vi "Dresden Edit Recipe(in).vi"() -> ()   [LabVIEW 2009] (continued)
                    n1981 = property on="R Single RF Interval length9" class="DigNum (strict)"("DisabledEnum"=w1077) -> ()  [unwired: 2 in, 2 out]
                  }
                }
              }
            }
            n1982 = case shown="False" w984 {
              frame #0 {
                w1926 = 0.0 ("R Cmb Ch2 Step1 Coating Power")
                w1927 = T5."Disabled and Grayed Out" ("Disabled")
                n1983 = local write "R Cmb Ch2 Step1 Coating Power"(w1926) -> ()
                n1984 = local write "R Cmb Ch3 Step1 Coating Power"(w1926) -> ()
                n1985 = local write "R Cmb Interval length 1"(w1926) -> ()
                n1986 = property on="R Cmb Ch3 Step1 Coating Power" class="DigNum (strict)"("DisabledEnum"=w1927) -> ()  [unwired: 2 in, 2 out]
                n1987 = property on="R Cmb Ch2 Step1 Coating Power" class="DigNum (strict)"("DisabledEnum"=w1927) -> ()  [unwired: 2 in, 2 out]
                n1988 = property on="R Cmb Interval length 1" class="DigNum (strict)"("DisabledEnum"=w1927) -> ()  [unwired: 2 in, 2 out]
              }
              frame #1 {
                w1928 = T5."Enabled" ("Disabled")
                n1989 = property on="R Cmb Ch3 Step1 Coating Power" class="DigNum (strict)"("DisabledEnum"=w1928) -> ()  [unwired: 2 in, 2 out]
                n1990 = property on="R Cmb Ch2 Step1 Coating Power" class="DigNum (strict)"("DisabledEnum"=w1928) -> ()  [unwired: 2 in, 2 out]
                n1991 = property on="R Cmb Interval length 1" class="DigNum (strict)"("DisabledEnum"=w1928) -> ()  [unwired: 2 in, 2 out]
              }
            }
            n1992 = case shown="True" "Calculate" {
              frame #0 {
              }
              frame #1 {
                n1993 = stacked-sequence {
                  frame #0 {
                    w1932 = 0.0 ("Lap")
                    n1994 = local read "R Minimum diameter"() -> (w1933:dbl)
                    n1995 = local write "Diameter"(w1933) -> ()
                    n1996 = local write "R  Total length"(w1932) -> ()
                    n1997 = local write "Lap"(w1932) -> ()
                  }
                  frame #1 {
                    n1998 = while {
                      stop <- w1936 stop-if-true
                      n1999 = local read "R Web thickness"() -> (w1946:dbl)
                      n2000 = Wait Until Next ms Multiple(millisecond multiple=u32 10) -> ()  [unwired: 1 out]
                      n2001 = Multiply(x=w1946, y=0.002) -> (x*y=w1945:dbl)
                      n2002 = local read "Lap"() -> (w1949:dbl)
                      n2003 = Increment(x=w1949) -> (x+1=→"Lap":dbl)
                      n2004 = Add(x="Diameter", y=w1945) -> (x+y=w1944:dbl)
                      n2005 = local write "Diameter"(w1944) -> ()
                      n2006 = local read "R Maximum diameter"() -> (w1937:dbl)
                      n2007 = local read "Diameter"() -> (w1934:dbl)
                      n2008 = Greater Or Equal?(x=w1934, y=w1937) -> (x >= y?=w1936:bool)
                      n2009 = local read "R  Total length"() -> (w1935:dbl)
                      n2010 = Multiply(x=w1934, y=3.141592653589793) -> (x*y=w1943:dbl)
                      n2011 = Divide(x=w1943, y=10.0) -> (x/y=w1940:dbl)
                      n2012 = Add(x=w1940, y=w1935) -> (x+y=→"R  Total length":dbl)
                    }
                  }
                }
              }
            }
            n2013 = case shown="False" "Power_single_rf_list_open" {
              frame #0 {
                n2014 = property on="Single_RF_power_power_tab" class="TabCtl (strict)"("Visible"=FALSE) -> ()  [unwired: 2 in, 2 out]
              }
              frame #1 {
                n2015 = property on="Single_RF_power_power_tab" class="TabCtl (strict)"("Visible"=TRUE) -> ()  [unwired: 2 in, 2 out]
              }
            }
            n2016 = local read "R Cmb Step6 Coating Power Active"() -> (w827:bool)
            n2017 = local read "R Cmb Step5 Coating Power Active"() -> (w828:bool)
            n2018 = local read "R Cmb Step7 Coating Power Active"() -> (w826:bool)
            n2019 = case shown="23" "R_Single RF_Mat_sel" {
              frame #0 {
              }
              frame #1 {
                n2020 = local write "R Single RF Target material"("Ag" ("R DC Target material")) -> ()
              }
              frame #2 {
                n2021 = local write "R Single RF Target material"("AgBr" ("R DC Target material")) -> ()
              }
              frame #3 {
                n2022 = local write "R Single RF Target material"("AgCl" ("R DC Target material")) -> ()
              }
              frame #4 {
                n2023 = local write "R Single RF Target material"("Al" ("R DC Target material")) -> ()
              }
              frame #5 {
                n2024 = local write "R Single RF Target material"("Al2O3" ("R DC Target material")) -> ()
              }
              frame #6 {
                n2025 = local write "R Single RF Target material"("As" ("R DC Target material")) -> ()
              }
              frame #7 {
                n2026 = local write "R Single RF Target material"("Au" ("R DC Target material")) -> ()
              }
              frame #8 {
                n2027 = local write "R Single RF Target material"("B" ("R DC Target material")) -> ()
              }
              frame #9 {
                n2028 = local write "R Single RF Target material"("Ba" ("R DC Target material")) -> ()
              }
              frame #10 {
                n2029 = local write "R Single RF Target material"("Be" ("R DC Target material")) -> ()
              }
              frame #11 {
                n2030 = local write "R Single RF Target material"("Bi" ("R DC Target material")) -> ()
              }
              frame #12 {
                n2031 = local write "R Single RF Target material"("Bi2O3" ("R DC Target material")) -> ()
              }
              frame #13 {
                n2032 = local write "R Single RF Target material"("C (Diamond)" ("R DC Target material")) -> ()
              }
              frame #14 {
                n2033 = local write "R Single RF Target material"("C (Graphite)" ("R DC Target material")) -> ()
              }
              frame #15 {
                n2034 = local write "R Single RF Target material"("Ca" ("R DC Target material")) -> ()
              }
              frame #16 {
                n2035 = local write "R Single RF Target material"("CaF" ("R DC Target material")) -> ()
              }
              frame #17 {
                n2036 = local write "R Single RF Target material"("Cd" ("R DC Target material")) -> ()
              }
              frame #18 {
                n2037 = local write "R Single RF Target material"("CdS" ("R DC Target material")) -> ()
              }
              frame #19 {
                n2038 = local write "R Single RF Target material"("CdSe" ("R DC Target material")) -> ()
              }
              frame #20 {
                n2039 = local write "R Single RF Target material"("CdTe" ("R DC Target material")) -> ()
              }
              frame #21 {
                n2040 = local write "R Single RF Target material"("CeF3" ("R DC Target material")) -> ()
              }
              frame #22 {
                n2041 = local write "R Single RF Target material"("CeO" ("R DC Target material")) -> ()
              }
              frame #23 {
                n2042 = local write "R Single RF Target material"("Cr" ("R DC Target material")) -> ()
              }
              frame #24 {
                n2043 = local write "R Single RF Target material"("Cr2O3" ("R DC Target material")) -> ()
              }
              frame #25 {
                n2044 = local write "R Single RF Target material"("Co" ("R DC Target material")) -> ()
              }
              frame #26 {
                n2045 = local write "R Single RF Target material"("Cu" ("R DC Target material")) -> ()
              }
              frame #27 {
                n2046 = local write "R Single RF Target material"("Cu2S (A)" ("R DC Target material")) -> ()
              }
              frame #28 {
                n2047 = local write "R Single RF Target material"("Cu2S (B)" ("R DC Target material")) -> ()
              }
              frame #29 {
                n2048 = local write "R Single RF Target material"("CuS" ("R DC Target material")) -> ()
              }
              frame #30 {
                n2049 = local write "R Single RF Target material"("Dy" ("R DC Target material")) -> ()
              }
              frame #31 {
                n2050 = local write "R Single RF Target material"("Er" ("R DC Target material")) -> ()
              }
              frame #32 {
                n2051 = local write "R Single RF Target material"("Fe" ("R DC Target material")) -> ()
              }
              frame #33 {
                n2052 = local write "R Single RF Target material"("Ga" ("R DC Target material")) -> ()
              }
              frame #34 {
                n2053 = local write "R Single RF Target material"("GaAs" ("R DC Target material")) -> ()
              }
              frame #35 {
                n2054 = local write "R Single RF Target material"("Gd" ("R DC Target material")) -> ()
              }
              frame #36 {
                n2055 = local write "R Single RF Target material"("Ge" ("R DC Target material")) -> ()
              }
              frame #37 {
                n2056 = local write "R Single RF Target material"("Hf" ("R DC Target material")) -> ()
              }
              frame #38 {
                n2057 = local write "R Single RF Target material"("HfO2" ("R DC Target material")) -> ()
              }
              frame #39 {
                n2058 = local write "R Single RF Target material"("Hg" ("R DC Target material")) -> ()
              }
              frame #40 {
                n2059 = local write "R Single RF Target material"("Ho" ("R DC Target material")) -> ()
              }
              frame #41 {
                n2060 = local write "R Single RF Target material"("In" ("R DC Target material")) -> ()
              }
              frame #42 {
                n2061 = local write "R Single RF Target material"("InSb" ("R DC Target material")) -> ()
              }
              frame #43 {
                n2062 = local write "R Single RF Target material"("In2O3" ("R DC Target material")) -> ()
              }
              frame #44 {
                n2063 = local write "R Single RF Target material"("Ir" ("R DC Target material")) -> ()
              }
              frame #45 {
                n2064 = local write "R Single RF Target material"("KCl" ("R DC Target material")) -> ()
              }
              frame #46 {
                n2065 = local write "R Single RF Target material"("La" ("R DC Target material")) -> ()
              }
              frame #47 {
                n2066 = local write "R Single RF Target material"("LaF3" ("R DC Target material")) -> ()
              }
              frame #48 {
                n2067 = local write "R Single RF Target material"("LaO3" ("R DC Target material")) -> ()
              }
              frame #49 {
                n2068 = local write "R Single RF Target material"("Li" ("R DC Target material")) -> ()
              }
              frame #50 {
                n2069 = local write "R Single RF Target material"("LiF" ("R DC Target material")) -> ()
              }
              frame #51 {
                n2070 = local write "R Single RF Target material"("Mg" ("R DC Target material")) -> ()
              }
              frame #52 {
                n2071 = local write "R Single RF Target material"("MgF2" ("R DC Target material")) -> ()
              }
              frame #53 {
                n2072 = local write "R Single RF Target material"("MgO" ("R DC Target material")) -> ()
              }
              frame #54 {
                n2073 = local write "R Single RF Target material"("Mn" ("R DC Target material")) -> ()
              }
              frame #55 {
                n2074 = local write "R Single RF Target material"("MnS" ("R DC Target material")) -> ()
              }
              frame #56 {
                n2075 = local write "R Single RF Target material"("Mo" ("R DC Target material")) -> ()
              }
              frame #57 {
                n2076 = local write "R Single RF Target material"("Na" ("R DC Target material")) -> ()
              }
              frame #58 {
                n2077 = local write "R Single RF Target material"("NaCl" ("R DC Target material")) -> ()
              }
              frame #59 {
                n2078 = local write "R Single RF Target material"("NdF3" ("R DC Target material")) -> ()
              }
              frame #60 {
                n2079 = local write "R Single RF Target material"("Nd2O3" ("R DC Target material")) -> ()
              }
              frame #61 {
                n2080 = local write "R Single RF Target material"("Ni" ("R DC Target material")) -> ()
              }
              frame #62 {
                n2081 = local write "R Single RF Target material"("Nb" ("R DC Target material")) -> ()
              }
              frame #63 {
                n2082 = local write "R Single RF Target material"("Nb2O5" ("R DC Target material")) -> ()
              }
              frame #64 {
                n2083 = local write "R Single RF Target material"("Pb" ("R DC Target material")) -> ()
              }
              frame #65 {
                n2084 = local write "R Single RF Target material"("PbS" ("R DC Target material")) -> ()
              }
              frame #66 {
                n2085 = local write "R Single RF Target material"("Pd" ("R DC Target material")) -> ()
              }
              frame #67 {
                n2086 = local write "R Single RF Target material"("Pt" ("R DC Target material")) -> ()
              }
              frame #68 {
                n2087 = local write "R Single RF Target material"("Re" ("R DC Target material")) -> ()
              }
              frame #69 {
                n2088 = local write "R Single RF Target material"("Rh" ("R DC Target material")) -> ()
              }
              frame #70 {
                n2089 = local write "R Single RF Target material"("Rb" ("R DC Target material")) -> ()
              }
              frame #71 {
                n2090 = local write "R Single RF Target material"("S" ("R DC Target material")) -> ()
              }
              frame #72 {
                n2091 = local write "R Single RF Target material"("Sb" ("R DC Target material")) -> ()
              }
              frame #73 {
                n2092 = local write "R Single RF Target material"("Sc" ("R DC Target material")) -> ()
              }
              frame #74 {
                n2093 = local write "R Single RF Target material"("Se" ("R DC Target material")) -> ()
              }
              frame #75 {
                n2094 = local write "R Single RF Target material"("Si" ("R DC Target material")) -> ()
              }
              frame #76 {
                n2095 = local write "R Single RF Target material"("SiO" ("R DC Target material")) -> ()
              }
              frame #77 {
                n2096 = local write "R Single RF Target material"("SiO2" ("R DC Target material")) -> ()
              }
              frame #78 {
                n2097 = local write "R Single RF Target material"("Sm" ("R DC Target material")) -> ()
              }
              frame #79 {
                n2098 = local write "R Single RF Target material"("Sn" ("R DC Target material")) -> ()
              }
              frame #80 {
                n2099 = local write "R Single RF Target material"("Ta" ("R DC Target material")) -> ()
              }
              frame #81 {
                n2100 = local write "R Single RF Target material"("Ta2O5" ("R DC Target material")) -> ()
              }
              frame #82 {
                n2101 = local write "R Single RF Target material"("Te" ("R DC Target material")) -> ()
              }
              frame #83 {
                n2102 = local write "R Single RF Target material"("Tb" ("R DC Target material")) -> ()
              }
              frame #84 {
                n2103 = local write "R Single RF Target material"("ThF4" ("R DC Target material")) -> ()
              }
              frame #85 {
                n2104 = local write "R Single RF Target material"("Ti" ("R DC Target material")) -> ()
              }
              frame #86 {
                n2105 = local write "R Single RF Target material"("TiO2" ("R DC Target material")) -> ()
              }
              frame #87 {
                n2106 = local write "R Single RF Target material"("TiO" ("R DC Target material")) -> ()
              }
              frame #88 {
                n2107 = local write "R Single RF Target material"("Tl" ("R DC Target material")) -> ()
              }
              frame #89 {
                n2108 = local write "R Single RF Target material"("U" ("R DC Target material")) -> ()
              }
              frame #90 {
                n2109 = local write "R Single RF Target material"("V" ("R DC Target material")) -> ()
              }
              frame #91 {
                n2110 = local write "R Single RF Target material"("W" ("R DC Target material")) -> ()
              }
              frame #92 {
                n2111 = local write "R Single RF Target material"("WC" ("R DC Target material")) -> ()
              }
              frame #93 {
                n2112 = local write "R Single RF Target material"("Y" ("R DC Target material")) -> ()
              }
              frame #94 {
                n2113 = local write "R Single RF Target material"("Y2O3" ("R DC Target material")) -> ()
              }
              frame #95 {
                n2114 = local write "R Single RF Target material"("Yb" ("R DC Target material")) -> ()
              }
              frame #96 {
                n2115 = local write "R Single RF Target material"("Zn" ("R DC Target material")) -> ()
              }
              frame #97 {
                n2116 = local write "R Single RF Target material"("ZnO" ("R DC Target material")) -> ()
              }
              frame #98 {
                n2117 = local write "R Single RF Target material"("ZnSe" ("R DC Target material")) -> ()
              }
              frame #99 {
                n2118 = local write "R Single RF Target material"("ZnS" ("R DC Target material")) -> ()
              }
              frame #100 {
                n2119 = local write "R Single RF Target material"("Zr" ("R DC Target material")) -> ()
              }
              frame #101 {
                n2120 = local write "R Single RF Target material"("ZrO2" ("R DC Target material")) -> ()
              }
              frame #102 {
                n2121 = local write "R Single RF Target material"("Si3N4" ("R DC Target material")) -> ()
              }
              frame #103 {
                n2122 = local write "R Single RF Target material"("ITO" ("R DC Target material")) -> ()
              }
              frame #104 {
                n2123 = local write "R Single RF Target material"("PbI2" ("R DC Target material")) -> ()
              }
            }
            n2124 = case shown="104" "R Cmb Ch3 Mat_sel" {
              frame #0 {
              }
              frame #1 {
                n2125 = local write "R Cmb Ch3 Target material"("Ag" ("R DC Target material")) -> ()
              }
              frame #2 {
                n2126 = local write "R Cmb Ch3 Target material"("AgBr" ("R DC Target material")) -> ()
              }
              frame #3 {
                n2127 = local write "R Cmb Ch3 Target material"("AgCl" ("R DC Target material")) -> ()
              }
              frame #4 {
                n2128 = local write "R Cmb Ch3 Target material"("Al" ("R DC Target material")) -> ()
              }
              frame #5 {
                n2129 = local write "R Cmb Ch3 Target material"("Al2O3" ("R DC Target material")) -> ()
              }
              frame #6 {
                n2130 = local write "R Cmb Ch3 Target material"("As" ("R DC Target material")) -> ()
              }
              frame #7 {
                n2131 = local write "R Cmb Ch3 Target material"("Au" ("R DC Target material")) -> ()
              }
              frame #8 {
                n2132 = local write "R Cmb Ch3 Target material"("B" ("R DC Target material")) -> ()
              }
              frame #9 {
                n2133 = local write "R Cmb Ch3 Target material"("Ba" ("R DC Target material")) -> ()
              }
              frame #10 {
                n2134 = local write "R Cmb Ch3 Target material"("Be" ("R DC Target material")) -> ()
              }
              frame #11 {
                n2135 = local write "R Cmb Ch3 Target material"("Bi" ("R DC Target material")) -> ()
              }
              frame #12 {
                n2136 = local write "R Cmb Ch3 Target material"("Bi2O3" ("R DC Target material")) -> ()
              }
              frame #13 {
                n2137 = local write "R Cmb Ch3 Target material"("C (Diamond)" ("R DC Target material")) -> ()
              }
              frame #14 {
                n2138 = local write "R Cmb Ch3 Target material"("C (Graphite)" ("R DC Target material")) -> ()
              }
              frame #15 {
                n2139 = local write "R Cmb Ch3 Target material"("Ca" ("R DC Target material")) -> ()
              }
              frame #16 {
                n2140 = local write "R Cmb Ch3 Target material"("CaF" ("R DC Target material")) -> ()
              }
              frame #17 {
                n2141 = local write "R Cmb Ch3 Target material"("Cd" ("R DC Target material")) -> ()
              }
              frame #18 {
                n2142 = local write "R Cmb Ch3 Target material"("CdS" ("R DC Target material")) -> ()
              }
              frame #19 {
                n2143 = local write "R Cmb Ch3 Target material"("CdSe" ("R DC Target material")) -> ()
              }
              frame #20 {
                n2144 = local write "R Cmb Ch3 Target material"("CdTe" ("R DC Target material")) -> ()
              }
              frame #21 {
                n2145 = local write "R Cmb Ch3 Target material"("CeF3" ("R DC Target material")) -> ()
              }
              frame #22 {
                n2146 = local write "R Cmb Ch3 Target material"("CeO" ("R DC Target material")) -> ()
              }
              frame #23 {
                n2147 = local write "R Cmb Ch3 Target material"("Cr" ("R DC Target material")) -> ()
              }
              frame #24 {
                n2148 = local write "R Cmb Ch3 Target material"("Cr2O3" ("R DC Target material")) -> ()
              }
              frame #25 {
                n2149 = local write "R Cmb Ch3 Target material"("Co" ("R DC Target material")) -> ()
              }
              frame #26 {
                n2150 = local write "R Cmb Ch3 Target material"("Cu" ("R DC Target material")) -> ()
              }
              frame #27 {
                n2151 = local write "R Cmb Ch3 Target material"("Cu2S (A)" ("R DC Target material")) -> ()
              }
              frame #28 {
                n2152 = local write "R Cmb Ch3 Target material"("Cu2S (B)" ("R DC Target material")) -> ()
              }
              frame #29 {
                n2153 = local write "R Cmb Ch3 Target material"("CuS" ("R DC Target material")) -> ()
              }
              frame #30 {
                n2154 = local write "R Cmb Ch3 Target material"("Dy" ("R DC Target material")) -> ()
              }
              frame #31 {
                n2155 = local write "R Cmb Ch3 Target material"("Er" ("R DC Target material")) -> ()
              }
              frame #32 {
                n2156 = local write "R Cmb Ch3 Target material"("Fe" ("R DC Target material")) -> ()
              }
              frame #33 {
                n2157 = local write "R Cmb Ch3 Target material"("Ga" ("R DC Target material")) -> ()
              }
              frame #34 {
                n2158 = local write "R Cmb Ch3 Target material"("GaAs" ("R DC Target material")) -> ()
              }
              frame #35 {
                n2159 = local write "R Cmb Ch3 Target material"("Gd" ("R DC Target material")) -> ()
              }
              frame #36 {
                n2160 = local write "R Cmb Ch3 Target material"("Ge" ("R DC Target material")) -> ()
              }
              frame #37 {
                n2161 = local write "R Cmb Ch3 Target material"("Hf" ("R DC Target material")) -> ()
              }
              frame #38 {
                n2162 = local write "R Cmb Ch3 Target material"("HfO2" ("R DC Target material")) -> ()
              }
              frame #39 {
                n2163 = local write "R Cmb Ch3 Target material"("Hg" ("R DC Target material")) -> ()
              }
              frame #40 {
                n2164 = local write "R Cmb Ch3 Target material"("Ho" ("R DC Target material")) -> ()
              }
              frame #41 {
                n2165 = local write "R Cmb Ch3 Target material"("In" ("R DC Target material")) -> ()
              }
              frame #42 {
                n2166 = local write "R Cmb Ch3 Target material"("InSb" ("R DC Target material")) -> ()
              }
              frame #43 {
                n2167 = local write "R Cmb Ch3 Target material"("In2O3" ("R DC Target material")) -> ()
              }
              frame #44 {
                n2168 = local write "R Cmb Ch3 Target material"("Ir" ("R DC Target material")) -> ()
              }
              frame #45 {
                n2169 = local write "R Cmb Ch3 Target material"("KCl" ("R DC Target material")) -> ()
              }
              frame #46 {
                n2170 = local write "R Cmb Ch3 Target material"("La" ("R DC Target material")) -> ()
              }
              frame #47 {
                n2171 = local write "R Cmb Ch3 Target material"("LaF3" ("R DC Target material")) -> ()
              }
              frame #48 {
                n2172 = local write "R Cmb Ch3 Target material"("LaO3" ("R DC Target material")) -> ()
              }
              frame #49 {
                n2173 = local write "R Cmb Ch3 Target material"("Li" ("R DC Target material")) -> ()
              }
              frame #50 {
                n2174 = local write "R Cmb Ch3 Target material"("LiF" ("R DC Target material")) -> ()
              }
              frame #51 {
                n2175 = local write "R Cmb Ch3 Target material"("Mg" ("R DC Target material")) -> ()
              }
              frame #52 {
                n2176 = local write "R Cmb Ch3 Target material"("MgF2" ("R DC Target material")) -> ()
              }
              frame #53 {
                n2177 = local write "R Cmb Ch3 Target material"("MgO" ("R DC Target material")) -> ()
              }
              frame #54 {
                n2178 = local write "R Cmb Ch3 Target material"("Mn" ("R DC Target material")) -> ()
              }
              frame #55 {
                n2179 = local write "R Cmb Ch3 Target material"("MnS" ("R DC Target material")) -> ()
              }
              frame #56 {
                n2180 = local write "R Cmb Ch3 Target material"("Mo" ("R DC Target material")) -> ()
              }
              frame #57 {
                n2181 = local write "R Cmb Ch3 Target material"("Na" ("R DC Target material")) -> ()
              }
              frame #58 {
                n2182 = local write "R Cmb Ch3 Target material"("NaCl" ("R DC Target material")) -> ()
              }
              frame #59 {
                n2183 = local write "R Cmb Ch3 Target material"("NdF3" ("R DC Target material")) -> ()
              }
              frame #60 {
                n2184 = local write "R Cmb Ch3 Target material"("Nd2O3" ("R DC Target material")) -> ()
              }
              frame #61 {
                n2185 = local write "R Cmb Ch3 Target material"("Ni" ("R DC Target material")) -> ()
              }
              frame #62 {
                n2186 = local write "R Cmb Ch3 Target material"("Nb" ("R DC Target material")) -> ()
              }
              frame #63 {
                n2187 = local write "R Cmb Ch3 Target material"("Nb2O5" ("R DC Target material")) -> ()
              }
              frame #64 {
                n2188 = local write "R Cmb Ch3 Target material"("Pb" ("R DC Target material")) -> ()
              }
              frame #65 {
                n2189 = local write "R Cmb Ch3 Target material"("PbS" ("R DC Target material")) -> ()
              }
              frame #66 {
                n2190 = local write "R Cmb Ch3 Target material"("Pd" ("R DC Target material")) -> ()
              }
              frame #67 {
                n2191 = local write "R Cmb Ch3 Target material"("Pt" ("R DC Target material")) -> ()
              }
              frame #68 {
                n2192 = local write "R Cmb Ch3 Target material"("Re" ("R DC Target material")) -> ()
              }
              frame #69 {
                n2193 = local write "R Cmb Ch3 Target material"("Rh" ("R DC Target material")) -> ()
              }
              frame #70 {
                n2194 = local write "R Cmb Ch3 Target material"("Rb" ("R DC Target material")) -> ()
              }
              frame #71 {
                n2195 = local write "R Cmb Ch3 Target material"("S" ("R DC Target material")) -> ()
              }
              frame #72 {
                n2196 = local write "R Cmb Ch3 Target material"("Sb" ("R DC Target material")) -> ()
              }
              frame #73 {
                n2197 = local write "R Cmb Ch3 Target material"("Sc" ("R DC Target material")) -> ()
              }
              frame #74 {
                n2198 = local write "R Cmb Ch3 Target material"("Se" ("R DC Target material")) -> ()
              }
              frame #75 {
                n2199 = local write "R Cmb Ch3 Target material"("Si" ("R DC Target material")) -> ()
              }
              frame #76 {
                n2200 = local write "R Cmb Ch3 Target material"("SiO" ("R DC Target material")) -> ()
              }
              frame #77 {
                n2201 = local write "R Cmb Ch3 Target material"("SiO2" ("R DC Target material")) -> ()
              }
              frame #78 {
                n2202 = local write "R Cmb Ch3 Target material"("Sm" ("R DC Target material")) -> ()
              }
              frame #79 {
                n2203 = local write "R Cmb Ch3 Target material"("Sn" ("R DC Target material")) -> ()
              }
              frame #80 {
                n2204 = local write "R Cmb Ch3 Target material"("Ta" ("R DC Target material")) -> ()
              }
              frame #81 {
                n2205 = local write "R Cmb Ch3 Target material"("Ta2O5" ("R DC Target material")) -> ()
              }
              frame #82 {
                n2206 = local write "R Cmb Ch3 Target material"("Te" ("R DC Target material")) -> ()
              }
              frame #83 {
                n2207 = local write "R Cmb Ch3 Target material"("Tb" ("R DC Target material")) -> ()
              }
              frame #84 {
                n2208 = local write "R Cmb Ch3 Target material"("ThF4" ("R DC Target material")) -> ()
              }
              frame #85 {
                n2209 = local write "R Cmb Ch3 Target material"("Ti" ("R DC Target material")) -> ()
              }
              frame #86 {
                n2210 = local write "R Cmb Ch3 Target material"("TiO2" ("R DC Target material")) -> ()
              }
              frame #87 {
                n2211 = local write "R Cmb Ch3 Target material"("TiO" ("R DC Target material")) -> ()
              }
              frame #88 {
                n2212 = local write "R Cmb Ch3 Target material"("Tl" ("R DC Target material")) -> ()
              }
              frame #89 {
                n2213 = local write "R Cmb Ch3 Target material"("U" ("R DC Target material")) -> ()
              }
              frame #90 {
                n2214 = local write "R Cmb Ch3 Target material"("V" ("R DC Target material")) -> ()
              }
              frame #91 {
                n2215 = local write "R Cmb Ch3 Target material"("W" ("R DC Target material")) -> ()
              }
              frame #92 {
                n2216 = local write "R Cmb Ch3 Target material"("WC" ("R DC Target material")) -> ()
              }
              frame #93 {
                n2217 = local write "R Cmb Ch3 Target material"("Y" ("R DC Target material")) -> ()
              }
              frame #94 {
                n2218 = local write "R Cmb Ch3 Target material"("Y2O3" ("R DC Target material")) -> ()
              }
              frame #95 {
                n2219 = local write "R Cmb Ch3 Target material"("Yb" ("R DC Target material")) -> ()
              }
              frame #96 {
